vi "Host3.vi"() -> ()   [LabVIEW 2025]
uses:
  <vilib>/numeric/Random Number (Range) U64.vi
  <vilib>/Analysis/baseanly.llb/Real Dot Product.vi
  <vilib>/Analysis/baseanly.llb/Real A x B.vi
  <vilib>/numeric/sub_Random U32.vi
  <vilib>/Analysis/Matrix/Numeric/Conversions/Matrix To Array - RM.vi
  <vilib>/FPGAPlugInAG/cRIO-9033/niLvFpga_Open_cRIO-9033.vi
  <vilib>/rvi/interface/common/dynamic/niFpgaDynamicAddResources.vi
  <vilib>/FPGAPlugInAG/Dynamic/niLvFpga_Reset_Dynamic.vi
  <vilib>/Utility/error.llb/Error Cluster From Error Code.vi
  <vilib>/rvi/errors/niLvFpgaAdjustHostInterfaceError.vi
  <vilib>/FPGAPlugInAG/Dynamic/niLvFpga_Run_Dynamic.vi
  <vilib>/FPGAPlugInAG/Dynamic/niLvFpga_Close_Dynamic.vi
  <vilib>/rvi/interface/nirviOpenFPGA/nirviOpenFPGA.xnode
  FPGA Bitfiles/dotplot9033_FPGATarget_Target2_yjTa3N87RjU.lvbitx
  Target2.vi
  <vilib>/rvi/interface/nirviMethod/nirviMethod.xnode
  <vilib>/rvi/interface/nirviReadWriteControl/nirviReadWriteControl.xnode
  <vilib>/rvi/interface/nirviCloseFPGA/nirviCloseFPGA.xnode
  <vilib>/rvi/errors/niLvFpgaMergeErrorWithErrorCode.vi
  <vilib>/Analysis/NI_AALBase.lvlib
  <vilib>/Analysis/Matrix/NI_Matrix.lvlib
  <vilib>/FPGAPlugInAG/Dynamic/niLvFpga_WriteFifo_Dynamic.vi
  <vilib>/FPGAPlugInAG/Dynamic/niLvFpga_ReadFifo_Dynamic.vi
  NiFpgaLv.dll
  <vilib>/rvi/interface/Simulation/niFpgaSimulationCallBeginRW.vi
panel:
  out "cr 2":fxp<+/-,32,16>[](array[numeric])
  out "element 4":fxp<+/-,32,16>
  out "element 3":fxp<+/-,32,16>
  out "element 2":fxp<+/-,32,16>
  out "element":fxp<+/-,32,16>
  out "interleaved array 2":fxp<+/-,32,16>[](array[numeric])
  out "interleaved array":fxp<+/-,32,16>[](array[numeric])
  out "Case Number":i16
  out "Numeric":i32
  out "appended array 2":fxp<+/-,32,16>[](array[numeric])
  out "appended array":fxp<+/-,32,16>[](array[numeric])
  out "cr":fxp<+/-,32,16>[](array[numeric])
  out "Elements Remaining":u32
  out "FIFO C Output":fxp<+/-,32,16>[](array[numeric])
  out "FIFO A Input":fxp<+/-,32,16>[](array[numeric])
  out "FIFO B Input":fxp<+/-,32,16>[](array[numeric])
  out "X * Y":fxp<+/-,64,32>
  out "elements in B":i32
  out "elements in A":i32
  out "sum of error":dbl
  out "C - FPGA code":fxp<+/-,32,16>[][](array[numeric])
  out "elements in C":i32
  out "C - Real":dbl[][](array[numeric])
  out "B":fxp<+/-,32,16>[][](array[numeric])
  out "A":fxp<+/-,32,16>[][](array[numeric])
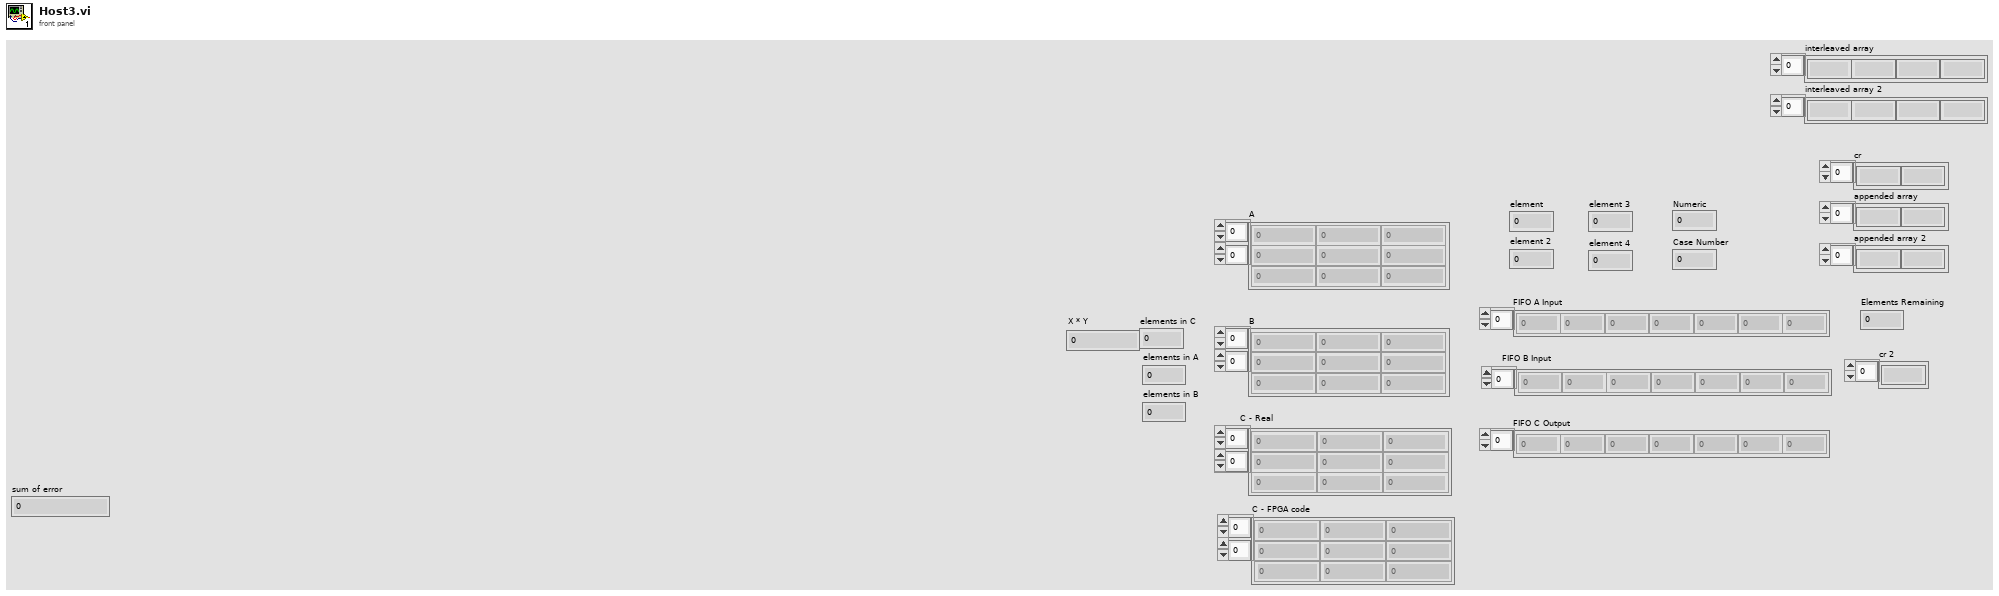
[diagram p1: front panel]
types:
  T1 = typedef "NI_Matrix.lvlib/RealMatrix.ctl" = dbl[][]
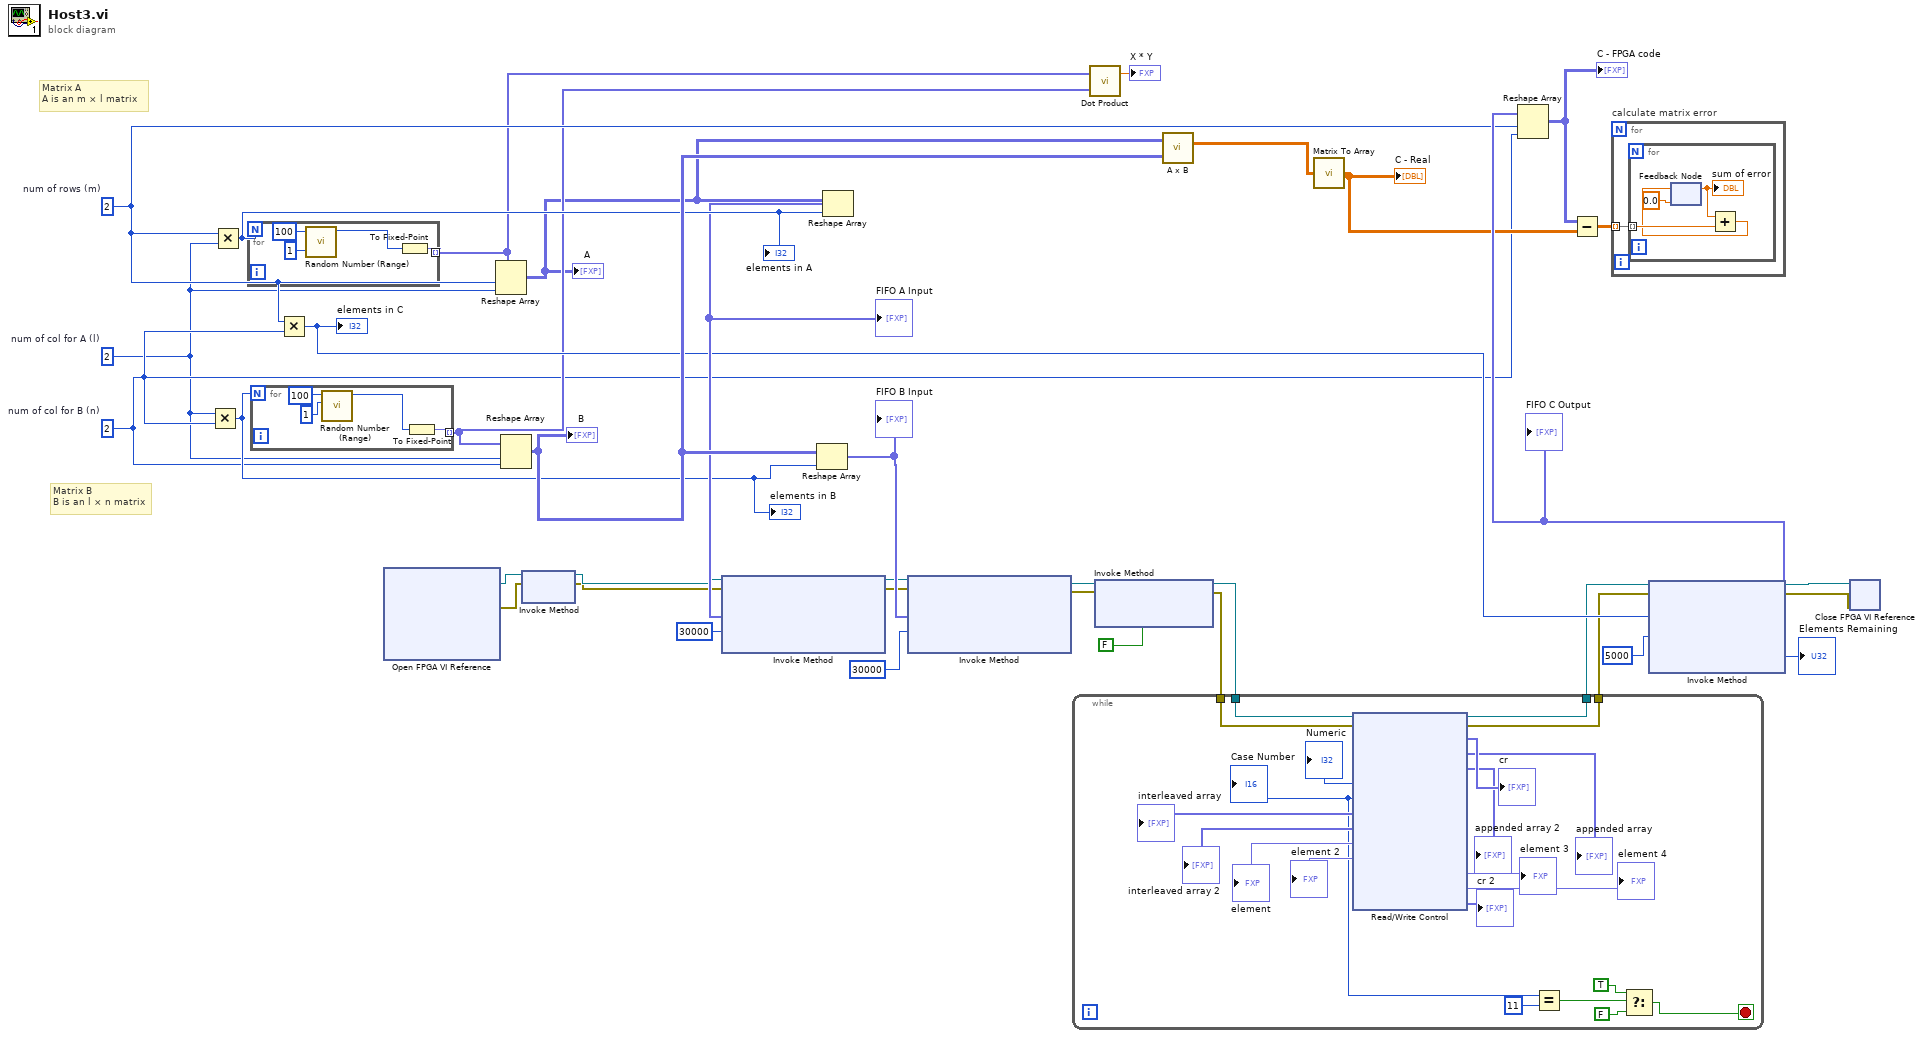
[diagram p0: block diagram]
diagram:
  w22 = 2  # num of col for B (n)
  w21 = 2  # num of col for A (l)
  w30 = 2  # num of rows (m)
  # "Matrix B\nB is an l × n matrix"
  # "Matrix A\nA is an m × l matrix"
  n1 = Multiply(x=w21, y=w22) -> (x*y=w27:i32)
  "elements in B" <- w27
  n2 = Multiply(x=w30, y=w21) -> (x*y=w35:i32)
  "elements in A" <- w35
  n3 = for {
    N: w35 -> [_]
    tunnel: [w41] -> w26 mode=indexing
    n4 = call-poly <vilib>:"Random Number (Range).vi"("lower bound (0)"=u64 1, "upper bound (100)"=u64 100) -> ("number"=w40:u64)  [unwired: 9 in]
    n5 = To Fixed-Point(number=w40) -> (fixed-point=w41:fxp<+,64,64>)  [unwired: 1 in]
  }
  n6 = for {
    N: w27 -> [_]
    tunnel: [w45] -> w25 mode=indexing
    n7 = call-poly <vilib>:"Random Number (Range).vi"("lower bound (0)"=u64 1, "upper bound (100)"=u64 100) -> ("number"=w42:u64)  [unwired: 9 in]
    n8 = To Fixed-Point(number=w42) -> (fixed-point=w45:fxp<+,64,64>)  [unwired: 1 in]
  }
  n9 = Multiply(x=w30, y=w22) -> (x*y=w28:i32)
  "elements in C" <- w28
  n10 = xnode "Open FPGA VI Reference"() -> ("FPGA VI Reference Out"=w19:refnum<k20>, "error out"=w16:errorcluster)  [unwired: 2 in]
  n11 = Reshape Array(w26, w30, w21) -> (w23:fxp<+,64,64>[][])
  "A" <- w23
  n12 = Reshape Array(w25, w21, w22) -> (w37:fxp<+,64,64>[][])
  "B" <- w37
  n13 = xnode "Invoke Method"("FPGA VI Reference In"=w19, "error in"=w16) -> ("FPGA VI Reference Out"=w18:refnum<k20>, "error out"=w17:errorcluster)
  n14 = Reshape Array(w37, w27) -> (w20:fxp<+,64,64>[])
  "FIFO B Input" <- w20
  n15 = Reshape Array(w23, w35) -> (w34:fxp<+,64,64>[])
  "FIFO A Input" <- w34
  n16 = xnode "Invoke Method"("FPGA VI Reference In"=w18, "error in"=w17, "Data"=w34, "Timeout (ms)"=30000) -> ("FPGA VI Reference Out"=w11:refnum<k20>, "error out"=w10:errorcluster)  [unwired: 1 out]
  n17 = xnode "Invoke Method"("FPGA VI Reference In"=w11, "error in"=w10, "Data"=w20, "Timeout (ms)"=30000) -> ("FPGA VI Reference Out"=w14:refnum<k20>, "error out"=w13:errorcluster)  [unwired: 1 out]
  n18 = call-poly <vilib>:"Dot Product.vi"("Y Vector"=w25, "X Vector"=w26) -> ("X * Y"=→"X * Y":dbl)  [unwired: 1 out]
  n19 = xnode "Invoke Method"("FPGA VI Reference In"=w14, "error in"=w13, "Wait Until Done (F)"=FALSE) -> ("FPGA VI Reference Out"=w4:refnum<k20>, "error out"=w3:errorcluster)
  n20 = while {
    tunnel: w4 -> [w56]
    tunnel: w3 -> [w55]
    tunnel: [w54] -> w2
    tunnel: [w53] -> w1
    stop <- w50 stop-if-true
    n21 = xnode "Read/Write Control"("FPGA VI Reference In"=w56, "error in"=w55) -> ("FPGA VI Reference Out"=w53:refnum<k20>, "error out"=w54:errorcluster, "cr"=→"cr":fxp<+/-,32,16>[], "appended array"=→"appended array":fxp<+/-,32,16>[], "appended array 2"=→"appended array 2":fxp<+/-,32,16>[], "Numeric"=→"Numeric":i32, "Case Number"=w52:i16, "interleaved array"=→"interleaved array":fxp<+/-,32,16>[], "interleaved array 2"=→"interleaved array 2":fxp<+/-,32,16>[], "element"=→"element":fxp<+/-,32,16>, "element 2"=→"element 2":fxp<+/-,32,16>, "element 3"=→"element 3":fxp<+/-,32,16>, "element 4"=→"element 4":fxp<+/-,32,16>, "cr 2"=→"cr 2":fxp<+/-,32,16>[])
    "Case Number" <- w52
    n22 = Equal?(x=w52, y=i16 11) -> (x = y?=w49:bool)
    n23 = Select(t=TRUE, s=w49, f=FALSE) -> (s? t:f=w50:bool)
  }
  n24 = call-poly <vilib>:"A x B.vi"("B"=w37, "A"=w23) -> ("A x B"=w36:T1)  [unwired: 1 out]
  n25 = call-poly <vilib>:"Matrix To Array.vi"("Real Matrix"=w36) -> ("Real 2D Array"=w29:dbl[][])
  "C - Real" <- w29
  n26 = xnode "Invoke Method"("FPGA VI Reference In"=w1, "error in"=w2, "Number of Elements"=w28, "Timeout (ms)"=5000) -> ("FPGA VI Reference Out"=w7:refnum<k20>, "error out"=w6:errorcluster, "Data"=w31:fxp<+/-,32,16>[], "Elements Remaining"=→"Elements Remaining":u32)
  "FIFO C Output" <- w31
  n27 = Reshape Array(w31, w30, w22) -> (w33:fxp<+/-,32,16>[][])
  "C - FPGA code" <- w33
  n28 = Subtract(x=w33, y=w29) -> (x-y=w32:dbl[][])
  n29 = for "calculate matrix error" {
    tunnel: w32 -> [w67] mode=indexing
    n30 = for {
      tunnel: w67 -> [w71] mode=indexing
      n31 = feedback #1(0.0) -> (w69:dbl)
      "sum of error" <- w69
      n32 = Add(x=w69, y=w71) -> (x+y=w70:dbl)
      n33 = feedback-in #1(w70) -> ()
    }
  }
  n34 = xnode "Close FPGA VI Reference"("FPGA VI Reference In"=w7, "error in"=w6) -> ()  [unwired: 1 out]
